vi "Ry.vi"(3 "Theta":T1=1.57 items=["pi"=3.14, "pi/2"=1.57], 4 "Wire in":T2) -> (1 "Wire out":T2)   [LabVIEW 2016]
uses:
  TypeDefs/Circuit Cluster.ctl
  Classes/GateAbst/GateAbst.lvclass
  TypeDefs/Phase selector.ctl
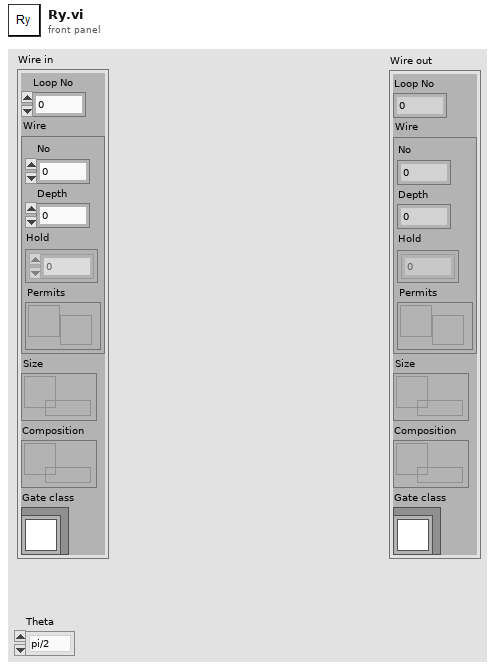
[diagram p1: front panel]
types:
  T1 = typedef "Phase selector.ctl" = dbl
  T2 = typedef "Circuit Cluster.ctl" = cluster{"Loop No":i32, "Wire":cluster{"No":i32, "Depth":i32, "Hold":i32[][], "Permits":refnum<notifier>}, "Size":refnum<queue>, "Composition":refnum<queue>, "Gate class":refnum<class "GateAbst.lvclass">}
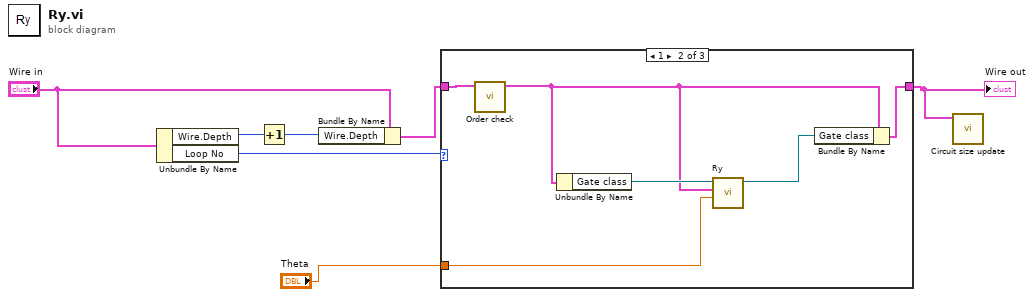
[diagram p0: block diagram]
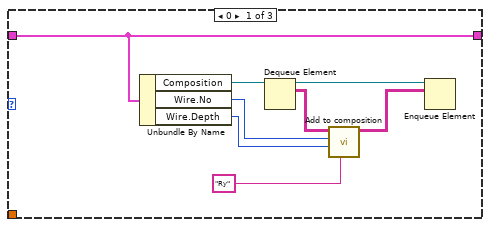
[diagram p2: hidden frame]
diagram:
  n1 = Unbundle By Name("Wire in") -> ("Wire.Depth"=w5:i32, "Loop No"=w1:i32)
  n2 = Increment(x=w5) -> (x+1=w6:i32)
  n3 = Bundle By Name(cluster="Wire in", "Wire.Depth"=w6) -> (w7:T2)
  n4 = case shown="1" w1 {
    tunnel: [w13 w20 w22] -> w2
    tunnel: w7 -> [w13 w18 w22]
    tunnel: "Theta" -> [_ w16 _]
    frame 0 {
      n5 = Unbundle By Name(w13) -> ("Composition"=w14:refnum<queue>, "Wire.No"=w9:i32, "Wire.Depth"=w8:i32)
      n6 = Dequeue Element(queue=w14) -> (queue out=w15:refnum<queue>, element=w10:string[][])  [unwired: 2 in, 2 out]
      n7 = call "Add to composition.vi"("Gate name"="Ry", "Wire depth"=w8, "Wire No"=w9, "Composition in"=w10) -> ("Composition out"=w11:string[][])  [unwired: 7 in]
      n8 = Enqueue Element(queue=w15, element=w11) -> ()  [unwired: 2 in, 3 out]
    }
    frame 1 {
      n9 = call "Order check.vi"("Wire in in"=w18) -> ("Wire out"=w17:T2)  [unwired: 10 in]
      n10 = Unbundle By Name(w17) -> ("Gate class"=w21:refnum<class "GateAbst.lvclass">)
      n11 = call-dynamic "Ry.vi"("Theta"=w16, "Wire in"=w17, "GateAbst in"=w21) -> ("GateAbst out"=w19:refnum<class "GateAbst.lvclass">)  [unwired: 7 in, 1 out]
      n12 = Bundle By Name(cluster=w17, "Gate class"=w19) -> (w20:T2)
    }
    frame Default {
    }
  }
  "Wire out" <- w2
  n13 = call "Circuit size update.vi"("Wire in"=w2) -> ()  [unwired: 11 in]
